vi "SLM Control.vi"() -> ()   [LabVIEW 2014]
uses:
  Controls/SLM General Settings.ctl
  Controls/Holo Controls.ctl
  <vilib>/Utility/xml.llb/Write to XML File(string).vi
  <vilib>/Utility/xml.llb/Read From XML File(string).vi
panel:
  in  "Load":bool
  in  "Save":bool
  in  "Exit":bool
  in  "Holo 1 (Doughnut)":T1={"Top Hat"=FALSE, "Modes"=[], "Vortex"=FALSE, "Clockwise"=FALSE, "X"=-200.0, "Y"=0.0, "Holo ON"=TRUE, "Scan"=FALSE, "Binary"=FALSE, "Binary Angle"=0.0} {"Modes"."Amplititute" step=0.05}
  out "Intensity Graph":u8[][](graph)
  in  "Holo 0 (Z)":T1={"Top Hat"=FALSE, "Modes"=[], "Vortex"=FALSE, "Clockwise"=FALSE, "X"=200.0, "Y"=0.0, "Holo ON"=TRUE, "Scan"=FALSE, "Binary"=FALSE, "Binary Angle"=0.0} {"Modes"."Amplititute" step=0.05}
  in  "General settings":T2={"Holo size (pixels)"=300, "Top hat radius"=0.5, "Number of modes"=20, "Bkg gradient X"=40.0, "Bkg gradient Y"=40.0, "Flat"=FALSE, "Mode Matrix"=1} {"Mode Matrix" items=["Unit Matrix", "Unit Matrix_AbbNames"]; "Top hat radius" min=0.0 max=0.99 step=0.05 format="%.3f"}
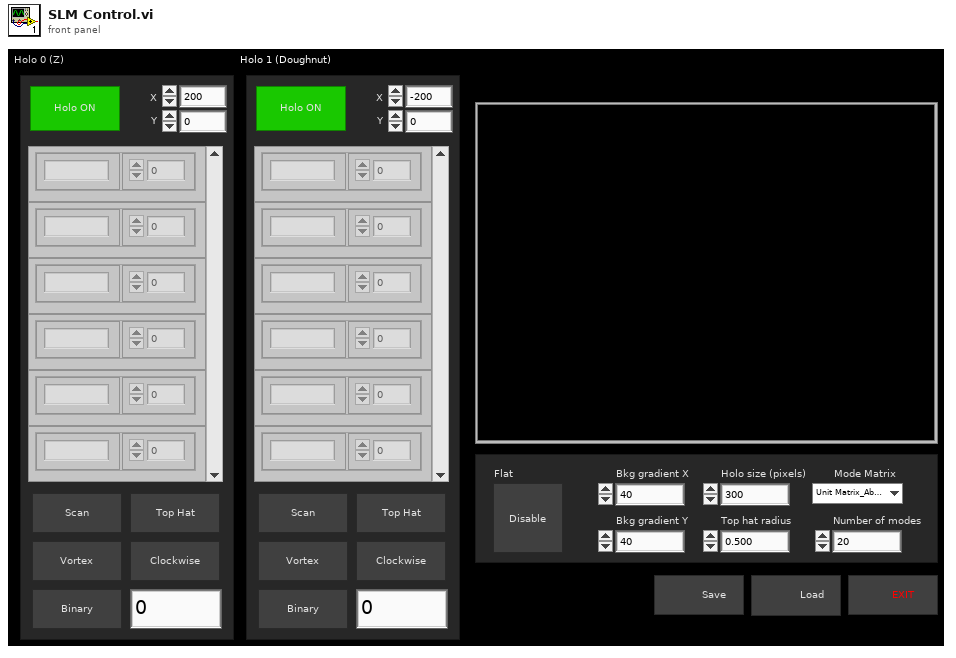
[diagram p1: front panel]
types:
  T1 = typedef "Holo Controls.ctl" = cluster{"Top Hat":bool, "Modes":cluster{"Mode ID":string, "Amplititute":dbl}[], "Vortex":bool, "Clockwise":bool, "X":dbl, "Y":dbl, "Holo ON":bool, "Scan":bool, "Binary":bool, "Binary Angle":dbl}
  T2 = typedef "SLM General Settings.ctl" = cluster{"Holo size (pixels)":i32, "Top hat radius":dbl, "Number of modes":i32, "Bkg gradient X":dbl, "Bkg gradient Y":dbl, "Flat":bool, "Mode Matrix":u16}
  T3 = cluster{"Holo size (pixels)":bool, "Top hat radius":bool, "Number of modes":bool, "Bkg gradient X":bool, "Bkg gradient Y":bool, "Flat":bool, "Mode Matrix":bool}
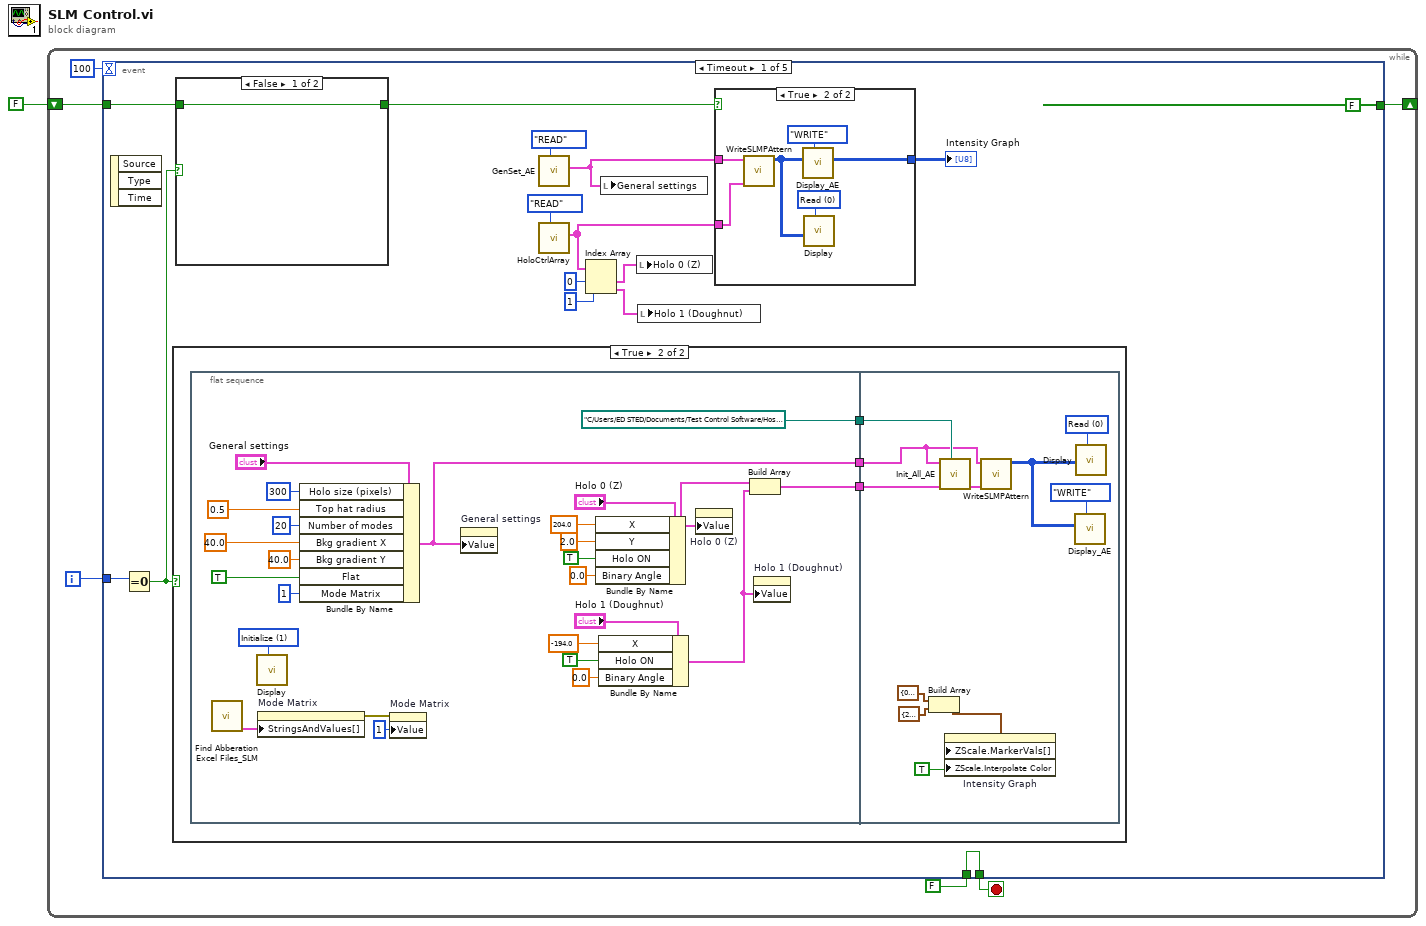
[diagram p0: block diagram]
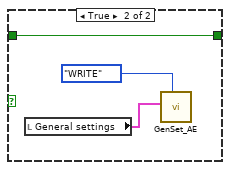
[diagram p2: hidden frame]
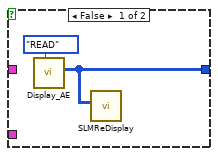
[diagram p3: hidden frame]
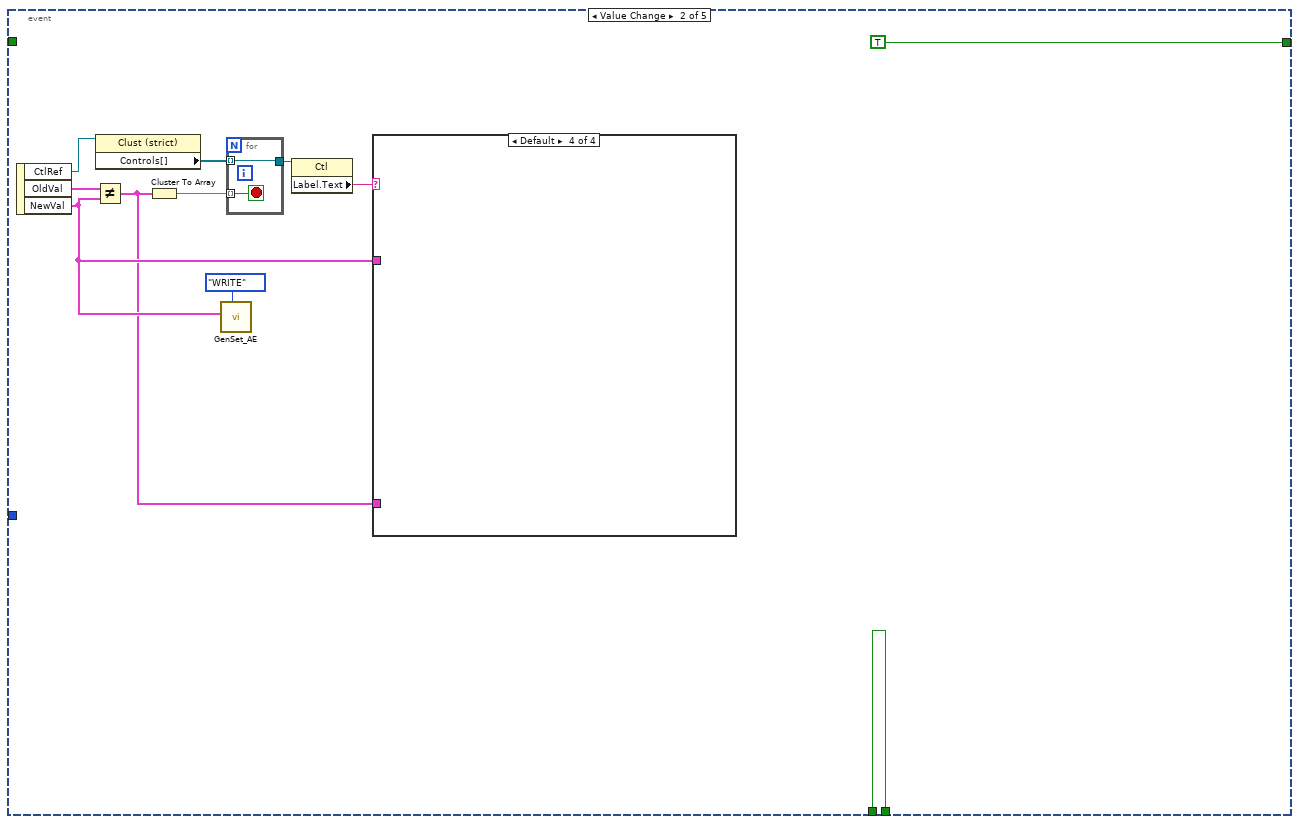
[diagram p5: hidden frame]
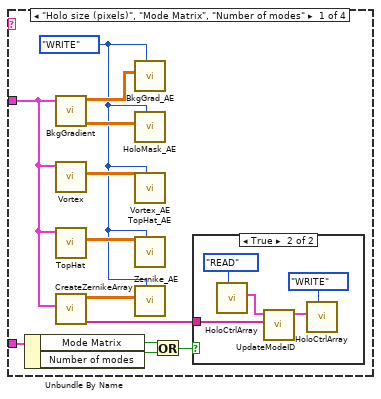
[diagram p6: hidden frame]
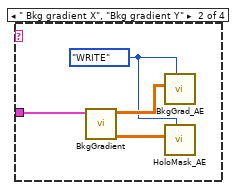
[diagram p8: hidden frame]
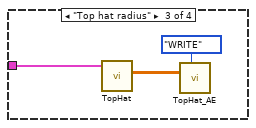
[diagram p9: hidden frame]
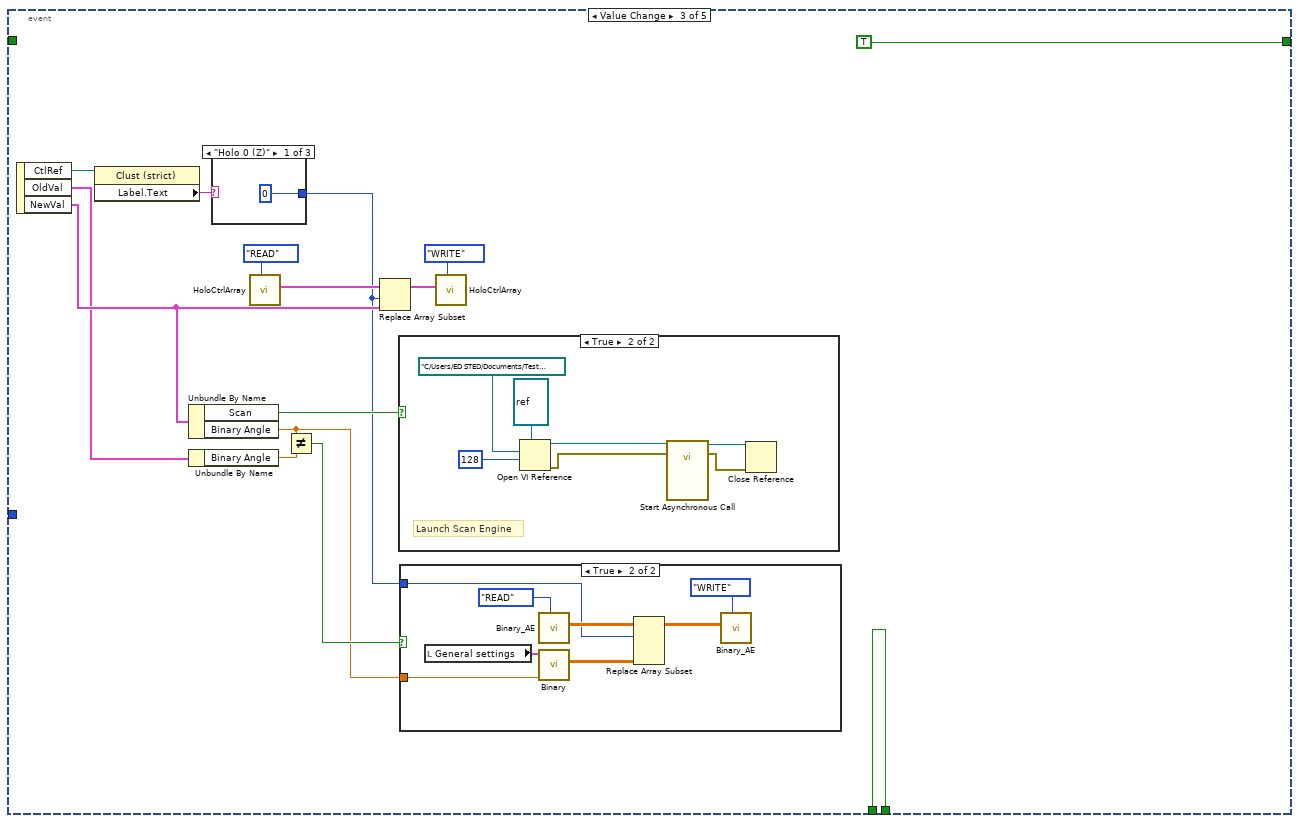
[diagram p10: hidden frame]
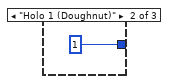
[diagram p13: hidden frame]
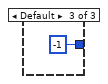
[diagram p14: hidden frame]
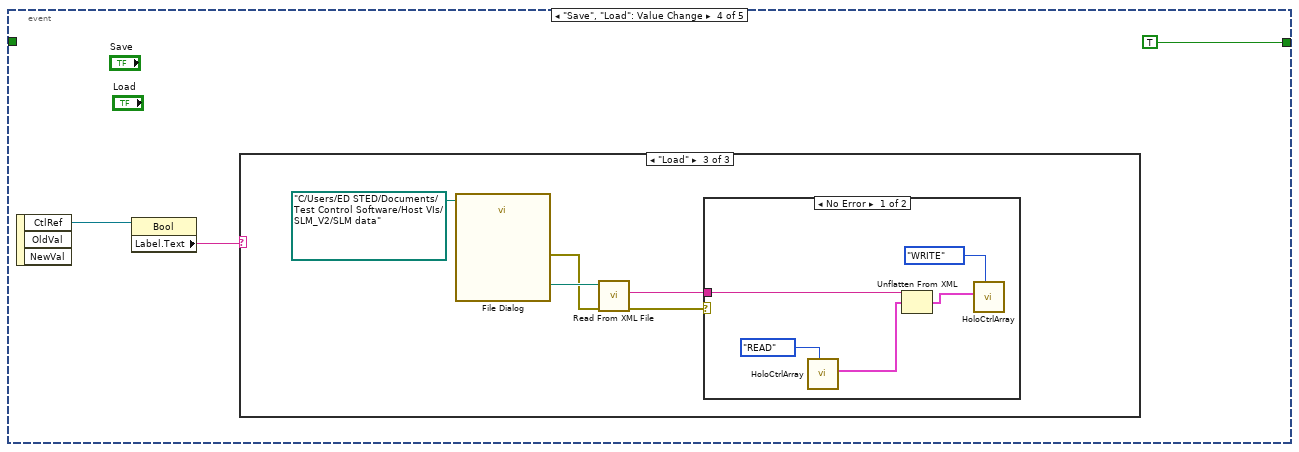
[diagram p15: hidden frame]
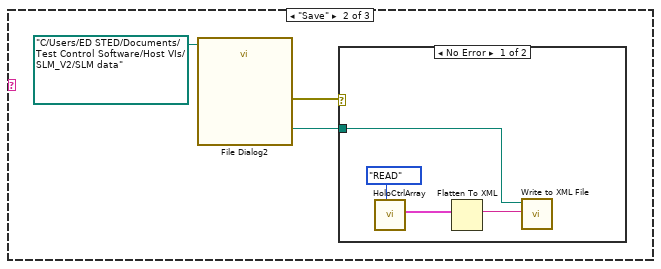
[diagram p17: hidden frame]
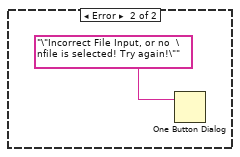
[diagram p18: hidden frame]
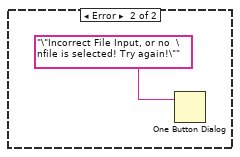
[diagram p19: hidden frame]
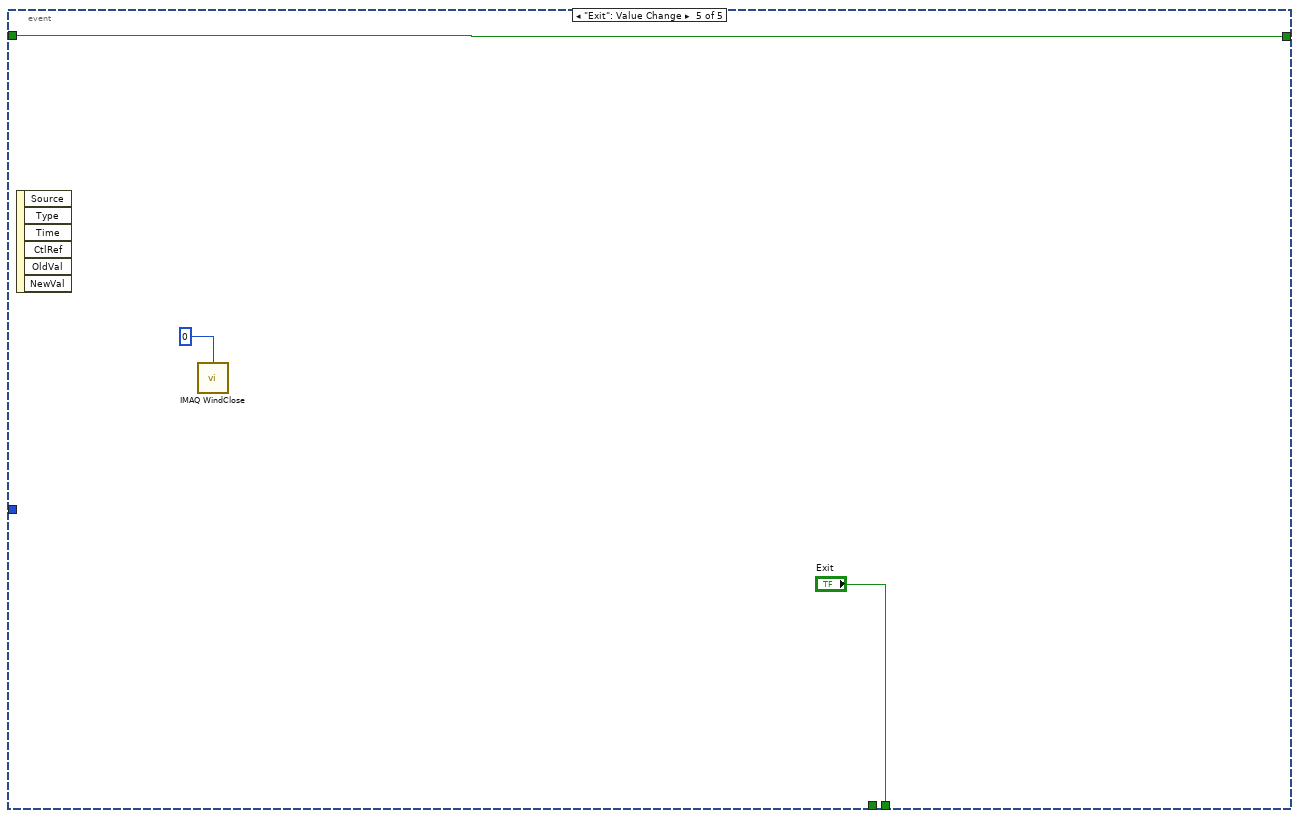
[diagram p20: hidden frame]
diagram:
  n1 = while {
    shift-right: [w4] -> _
    shift-left: FALSE -> [w5]
    i -> [w6]
    stop <- w3 stop-if-true
    n2 = event shown="[0] Timeout" {
      selector: _ -> [_ _ _ _ _]
      dyn-events: _ -> [_ _ _ _ _]
      timeout: 100 -> [_ _ _ _ _]
      tunnel: w6 -> [w22 _ _ _ _]
      tunnel: w5 -> [w10 _ _ _ w168]
      tunnel: [FALSE TRUE TRUE TRUE w168] -> w4
      tunnel: [w11 w76 w119 _ "Exit"] -> w3
      tunnel: FALSE -> [w11 w76 w119 _ _]
      event Timeout {
        n3 = event-data() -> ()  [unwired: 1 in, 3 out]
        n4 = Equal To 0?(x=w22) -> (x = 0?=w8:bool)
        n5 = case shown="True" w8 {
          frame False {
          }
          frame True {
            n6 = flat-sequence {
              tunnel: [w43] -> w37
              tunnel: [w59] -> w36
              tunnel: [path "C:/Users/ED STED/Documents/Test Control Software/Host VIs/SLM_V2/Flatness Correction LSH0701019/CAL_LSH0701019_770nm.bmp" ("Flat File Path")] -> w35
              tunnel: w37 -> [w66]
              tunnel: w36 -> [w74]
              tunnel: w35 -> [w71]
              frame #0 {
                w60 = u16 1 items=["Read", "Initialize"] ("Action")
                n7 = call "Find Abberation Excel Files_SLM.vi"() -> ("Ring Menu"=w63:cluster{"result string":string, i32}[])  [unwired: 10 in, 1 out]
                n8 = call "Display.vi"("Action"=w60) -> ()  [unwired: 10 in, 1 out]
                n9 = property on="Mode Matrix" class="Ring (strict)"("StringsAndValues[]"=w63) -> (error out=w62:errorcluster)  [unwired: 2 in, 1 out]
                n10 = Bundle By Name(cluster="General settings", "Holo size (pixels)"=300, "Top hat radius"=0.5, "Number of modes"=20, "Bkg gradient X"=40.0, "Bkg gradient Y"=40.0, "Flat"=TRUE, "Mode Matrix"=u16 1) -> (w43:T2)
                n11 = property on="Mode Matrix" class="Ring (strict)"(error in=w62, "Value"=u16 1) -> ()  [unwired: 1 in, 2 out]
                n12 = property on="General settings" class="Clust (strict)"("Value"=w43) -> ()  [unwired: 2 in, 2 out]
                n13 = Bundle By Name(cluster="Holo 0 (Z)", "X"=204.0, "Y"=2.0, "Holo ON"=TRUE, "Binary Angle"=0.0) -> (w47:T1)
                n14 = Bundle By Name(cluster="Holo 1 (Doughnut)", "X"=-194.0, "Holo ON"=TRUE, "Binary Angle"=0.0) -> (w44:T1)
                n15 = property on="Holo 0 (Z)" class="Clust (strict)"("Value"=w47) -> ()  [unwired: 2 in, 2 out]
                n16 = Build Array(w47, w44) -> (w59:T1[])
                n17 = property on="Holo 1 (Doughnut)" class="Clust (strict)"("Value"=w44) -> ()  [unwired: 2 in, 2 out]
              }
              frame #1 {
                w73 = u16 0 items=["Read", "Initialize"] ("Action")
                n18 = Build Array(cluster{dbl, u32} {0.0, 0}, cluster{dbl, u32} {255.0, 16448250}) -> (w67:cluster{dbl, u32}[])
                n19 = call "Init_All_AE.vi"("Flat File Path"=w71, "HoloArray In"=w74, "General settings"=w66) -> ("Holo Array Out"=w72:T1[])  [unwired: 8 in]
                n20 = property on="Intensity Graph" class="IntGraph (strict)"("ZScale.MarkerVals[]"=w67, "ZScale.Interpolate Color"=TRUE ("Z Scale.Interpolate Color")) -> ()  [unwired: 2 in, 2 out]
                n21 = call "WriteSLMPAttern.vi"("Holo Array"=w72, "General settings"=w66) -> ("Display Array"=w64:u8[][])  [unwired: 9 in]
                n22 = call "Display_AE.vi"("Action"=enum16{"READ", "WRITE"}."WRITE", "Display Array In"=w64) -> ()  [unwired: 9 in, 1 out]
                n23 = call "Display.vi"("Action"=w73, "displayed matrix"=w64) -> ()  [unwired: 9 in, 1 out]
              }
            }
          }
        }
        n24 = case shown="False" w8 {
          tunnel: w10 -> [w23 w26]
          tunnel: [w23 w26] -> w9
          frame False {
          }
          frame True {
            n25 = local read "General settings"() -> (w24:T2)
            n26 = call "GenSet_AE.vi"("Enum"=enum16{"READ", "WRITE"}."WRITE", "General settings"=w24) -> ()  [unwired: 9 in, 1 out]
          }
        }
        n27 = call "GenSet_AE.vi"("Enum"=enum16{"READ", "WRITE"}."READ") -> ("General settings Out"=w18:T2)  [unwired: 10 in]
        n28 = call "HoloCtrlArray.vi"("Action"=enum16{"READ", "WRITE"}."READ") -> ("Holo Array Out"=w17:T1[])  [unwired: 10 in]
        n29 = Index Array(array=w17, index #1=0 ("index"), index #2=1 ("index")) -> (element #1=w16:T1, element #2=w15:T1)
        n30 = local write "General settings"(w18) -> ()
        n31 = local write "Holo 0 (Z)"(w16) -> ()
        n32 = local write "Holo 1 (Doughnut)"(w15) -> ()
        n33 = case shown="True" w9 {
          tunnel: w18 -> [_ w34]
          tunnel: w17 -> [_ w33]
          tunnel: [w27 w29] -> w12
          frame False {
            n34 = call "Display_AE.vi"("Action"=enum16{"READ", "WRITE"}."READ") -> ("Display Array Out"=w27:u8[][])  [unwired: 10 in]
            n35 = call "SLMReDisplay.vi"("displayed matrix"=w27) -> ()  [unwired: 11 in]
          }
          frame True {
            w32 = u16 0 items=["Read", "Initialize"] ("Action")
            n36 = call "WriteSLMPAttern.vi"("Holo Array"=w33, "General settings"=w34) -> ("Display Array"=w31:u8[][])  [unwired: 9 in]
            n37 = call "Display_AE.vi"("Action"=enum16{"READ", "WRITE"}."WRITE", "Display Array In"=w31) -> ("Display Array Out"=w29:u8[][])  [unwired: 9 in]
            n38 = call "Display.vi"("Action"=w32, "displayed matrix"=w31) -> ()  [unwired: 9 in, 1 out]
          }
        }
        "Intensity Graph" <- w12
      }
      event Value Change {
        n39 = event-data() -> ("CtlRef"=w84:refnum<vi>, "OldVal"=w85:T2, "NewVal"=w77:T2)  [unwired: 1 in]
        n40 = Not Equal?(x=w85, y=w77) -> (x != y?=w75:T3)
        n41 = property class="Clust (strict)"(reference=w84) -> ("Controls[]"=w83:refnum<vi>[])  [unwired: 1 in, 2 out]
        n42 = Cluster To Array(cluster=w75) -> (array=w82:bool[])
        n43 = call "GenSet_AE.vi"("Enum"=enum16{"READ", "WRITE"}."WRITE", "General settings"=w77) -> ()  [unwired: 9 in, 1 out]
        n44 = for {
          tunnel: [w111] -> w81
          tunnel: w83 -> [w111] mode=indexing
          tunnel: w82 -> [w110] mode=indexing
          stop <- w110 stop-if-true
        }
        n45 = property class="Ctl"(reference=w81) -> ("Label.Text"=w80:string)  [unwired: 1 in, 2 out]
        n46 = case shown="Default" w80 {
          tunnel: w77 -> [w91 w103 w109 _]
          tunnel: w75 -> [w89 _ _ _]
          frame "Holo size (pixels)", "Mode Matrix", "Number of modes" {
            w90 = enum16{"READ", "WRITE"}."WRITE" ("Action")
            n47 = Unbundle By Name(w89) -> ("Mode Matrix"=w88:bool, "Number of modes"=w87:bool)
            n48 = call "BkgGradient.vi"("General settings"=w91) -> ("Holo mask"=w96:dbl[][], "gradient"=w97:dbl[][])  [unwired: 9 in]
            n49 = call "Vortex.vi"("General settings"=w91) -> ("Vortex"=w94:dbl[][])  [unwired: 10 in]
            n50 = call "TopHat.vi"("General settings"=w91) -> ("TopHat"=w95:dbl[][])  [unwired: 10 in]
            n51 = call "CreateZernikeArray.vi"("General settings"=w91) -> ("Mode IDs"=w92:string[], "Modes Out"=w93:dbl[][][])  [unwired: 9 in]
            n52 = call "BkgGrad_AE.vi"("Action"=w90, "BkgGrad In"=w97) -> ()  [unwired: 9 in, 1 out]
            n53 = call "HoloMask_AE.vi"("Action"=w90, "HoloMask In"=w96) -> ()  [unwired: 9 in, 1 out]
            n54 = call "Vortex_AE.vi"("Action"=w90, "Vortex In"=w94) -> ()  [unwired: 9 in, 1 out]
            n55 = call "TopHat_AE.vi"("Action"=w90, "TopHat In"=w95) -> ()  [unwired: 9 in, 1 out]
            n56 = call "Zernike_AE.vi"("Action"=w90, "Zernike In"=w93) -> ()  [unwired: 9 in, 1 out]
            n57 = Or(x=w88, y=w87) -> (x .or. y?=w86:bool)
            n58 = case shown="True" w86 {
              tunnel: w92 -> [_ w102]
              frame False {
              }
              frame True {
                n59 = call "HoloCtrlArray.vi"("Action"=enum16{"READ", "WRITE"}."READ") -> ("Holo Array Out"=w101:T1[])  [unwired: 10 in]
                n60 = call "UpdateModeID.vi"("Mode IDs"=w102, "Array in"=w101) -> ("Array out"=w98:T1[])  [unwired: 9 in]
                n61 = call "HoloCtrlArray.vi"("Action"=enum16{"READ", "WRITE"}."WRITE", "Holo Array In"=w98) -> ()  [unwired: 9 in, 1 out]
              }
            }
          }
          frame " Bkg gradient X", "Bkg gradient Y" {
            w104 = enum16{"READ", "WRITE"}."WRITE" ("Action")
            n62 = call "BkgGradient.vi"("General settings"=w103) -> ("Holo mask"=w105:dbl[][], "gradient"=w106:dbl[][])  [unwired: 9 in]
            n63 = call "BkgGrad_AE.vi"("Action"=w104, "BkgGrad In"=w106) -> ()  [unwired: 9 in, 1 out]
            n64 = call "HoloMask_AE.vi"("Action"=w104, "HoloMask In"=w105) -> ()  [unwired: 9 in, 1 out]
          }
          frame "Top hat radius" {
            n65 = call "TopHat.vi"("General settings"=w109) -> ("TopHat"=w108:dbl[][])  [unwired: 10 in]
            n66 = call "TopHat_AE.vi"("Action"=enum16{"READ", "WRITE"}."WRITE", "TopHat In"=w108) -> ()  [unwired: 9 in, 1 out]
          }
          frame Default {
          }
        }
      }
      event Value Change {
        n67 = event-data() -> ("CtlRef"=w123:refnum<vi>, "OldVal"=w116:T1, "NewVal"=w118:T1)  [unwired: 1 in]
        n68 = property class="Clust (strict)"(reference=w123) -> ("Label.Text"=w122:string)  [unwired: 1 in, 2 out]
        n69 = Unbundle By Name(w118) -> ("Scan"=w117:bool, "Binary Angle"=w113:dbl)
        n70 = Unbundle By Name(w116) -> ("Binary Angle"=w115:dbl)
        n71 = case shown="\"Holo 0 (Z)\"" w122 {
          tunnel: [0 1 -1] -> w112
          frame "Holo 0 (Z)" {
          }
          frame "Holo 1 (Doughnut)" {
          }
          frame Default {
          }
        }
        n72 = call "HoloCtrlArray.vi"("Action"=enum16{"READ", "WRITE"}."READ") -> ("Holo Array Out"=w124:T1[])  [unwired: 10 in]
        n73 = Not Equal?(x=w113, y=w115) -> (x != y?=w114:bool)
        n74 = Replace Array Subset(array=w124, new element=w118, index=w112) -> (w120:T1[])
        n75 = case shown="True" w117 {
          frame False {
          }
          frame True {
            # "Launch Scan Engine"
            n76 = Open VI Reference(type specifier VI Refnum (for type only)=refnum<vi> refnum, vi path=path "C:/Users/ED STED/Documents/Test Control Software/Host VIs/SLM_V2/Scan/ScanMode_SLM.vi", options=128) -> (vi reference=w136:refnum<vi>, error out=w135:errorcluster)  [unwired: 3 in]
            n77 = call-by-ref "Start Asynchronous Call"(reference=w136, error in=w135) -> (reference out=w138:refnum<vi>, error out=w137:errorcluster)  [unwired: 12 in]
            n78 = Close Reference(reference=w138, error in (no error)=w137) -> ()  [unwired: 1 out]
          }
        }
        n79 = case shown="True" w114 {
          tunnel: w113 -> [_ w133]
          tunnel: w112 -> [_ w127]
          frame False {
          }
          frame True {
            n80 = local read "General settings"() -> (w134:T2)
            n81 = call "Binary_AE.vi"("Action"=enum16{"READ", "WRITE"}."READ") -> ("BINARY Out"=w131:dbl[][][])  [unwired: 10 in]
            n82 = call "Binary.vi"("Angle"=w133, "General settings"=w134) -> ("Binary"=w130:dbl[][])  [unwired: 9 in]
            n83 = Replace Array Subset(array=w131, new element=w130, index (dim 0)=w127) -> (w128:dbl[][][])  [unwired: 2 in]
            n84 = call "Binary_AE.vi"("Action"=enum16{"READ", "WRITE"}."WRITE", "BINARY In"=w128) -> ()  [unwired: 9 in, 1 out]
          }
        }
        n85 = call "HoloCtrlArray.vi"("Action"=enum16{"READ", "WRITE"}."WRITE", "Holo Array In"=w120) -> ()  [unwired: 9 in, 1 out]
      }
      event "Save", "Load": Value Change {
        n86 = event-data() -> ("CtlRef"=w147:refnum<vi>)  [unwired: 1 in, 2 out]
        n87 = property class="Bool"(reference=w147) -> ("Label.Text"=w146:string)  [unwired: 1 in, 2 out]
        n88 = case shown="\"Load\"" w146 {
          frame Default {
          }
          frame "Save" {
            n89 = call "File Dialog2"("start path"=path "C:/Users/ED STED/Documents/Test Control Software/Host VIs/SLM_V2/SLM data") -> ("selected path"=w149:path, "error out"=w148:errorcluster)  [unwired: 11 in, 2 out]
            n90 = case shown="No Error" w148 {
              tunnel: w149 -> [w151 _]
              frame No Error {
                n91 = call "HoloCtrlArray.vi"("Action"=enum16{"READ", "WRITE"}."READ") -> ("Holo Array Out"=w153:T1[])  [unwired: 10 in]
                n92 = Flatten To XML(anything=w153) -> (xml string=w152:string)
                n93 = call-poly <vilib>:"Write to XML File.vi"("XML Input"=w152, "XML File Path"=w151) -> ()  [unwired: 7 in, 3 out]
              }
              frame Error {
                n94 = One Button Dialog(message="\"Incorrect File Input, or no  \nfile is selected! Try again!\"") -> ()  [unwired: 1 in, 1 out]
              }
            }
          }
          frame "Load" {
            n95 = call "File Dialog"("start path"=path "C:/Users/ED STED/Documents/Test Control Software/Host VIs/SLM_V2/SLM data") -> ("selected path"=w159:path, "error out"=w156:errorcluster)  [unwired: 11 in, 2 out]
            n96 = call-poly <vilib>:"Read From XML File.vi"("error in (no error)"=w156, "XML File Path"=w159) -> ("error out"=w157:errorcluster, "XML Elements"=w160:string)  [unwired: 7 in, 1 out]
            n97 = case shown="No Error" w157 {
              tunnel: w160 -> [w165 _]
              frame No Error {
                n98 = call "HoloCtrlArray.vi"("Action"=enum16{"READ", "WRITE"}."READ") -> ("Holo Array Out"=w163:T1[])  [unwired: 10 in]
                n99 = Unflatten From XML(xml string=w165, type=w163) -> (value=w162:T1[])  [unwired: 1 in, 1 out]
                n100 = call "HoloCtrlArray.vi"("Action"=enum16{"READ", "WRITE"}."WRITE", "Holo Array In"=w162) -> ()  [unwired: 9 in, 1 out]
              }
              frame Error {
                n101 = One Button Dialog(message="\"Incorrect File Input, or no  \nfile is selected! Try again!\"") -> ()  [unwired: 1 in, 1 out]
              }
            }
          }
        }
      }
      event "Exit": Value Change {
        n102 = event-data() -> ()  [unwired: 1 in, 6 out]
        n103 = call "IMAQ WindClose"("Window Number (0...15)"=0) -> ()  [unwired: 2 in, 4 out]
      }
    }
  }
